vi "SUB_SFCS_SEND_RFPI_IPEI_INFO.vi"(0 "URL":string, 1 "SN":string, 2 "Stage":string, 3 "InfoName":string, 4 "RFID_ID":string="246812345") -> (5 "Pass ?":bool, 6 "All output":string)   [LabVIEW 2011]
uses:
  data/MCSDLL.dll
panel:
  out "OUT1":string
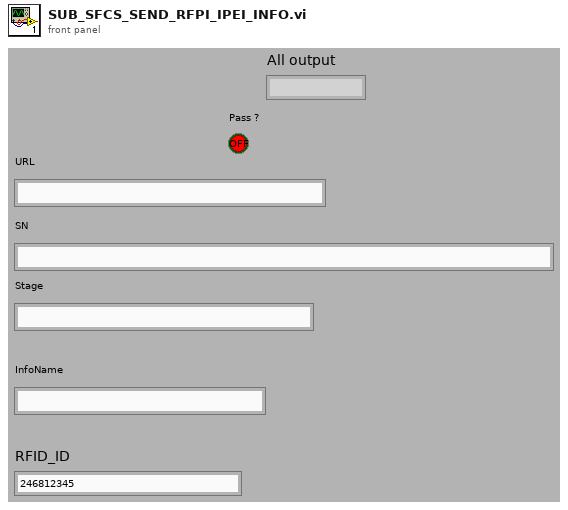
[diagram p1: front panel]
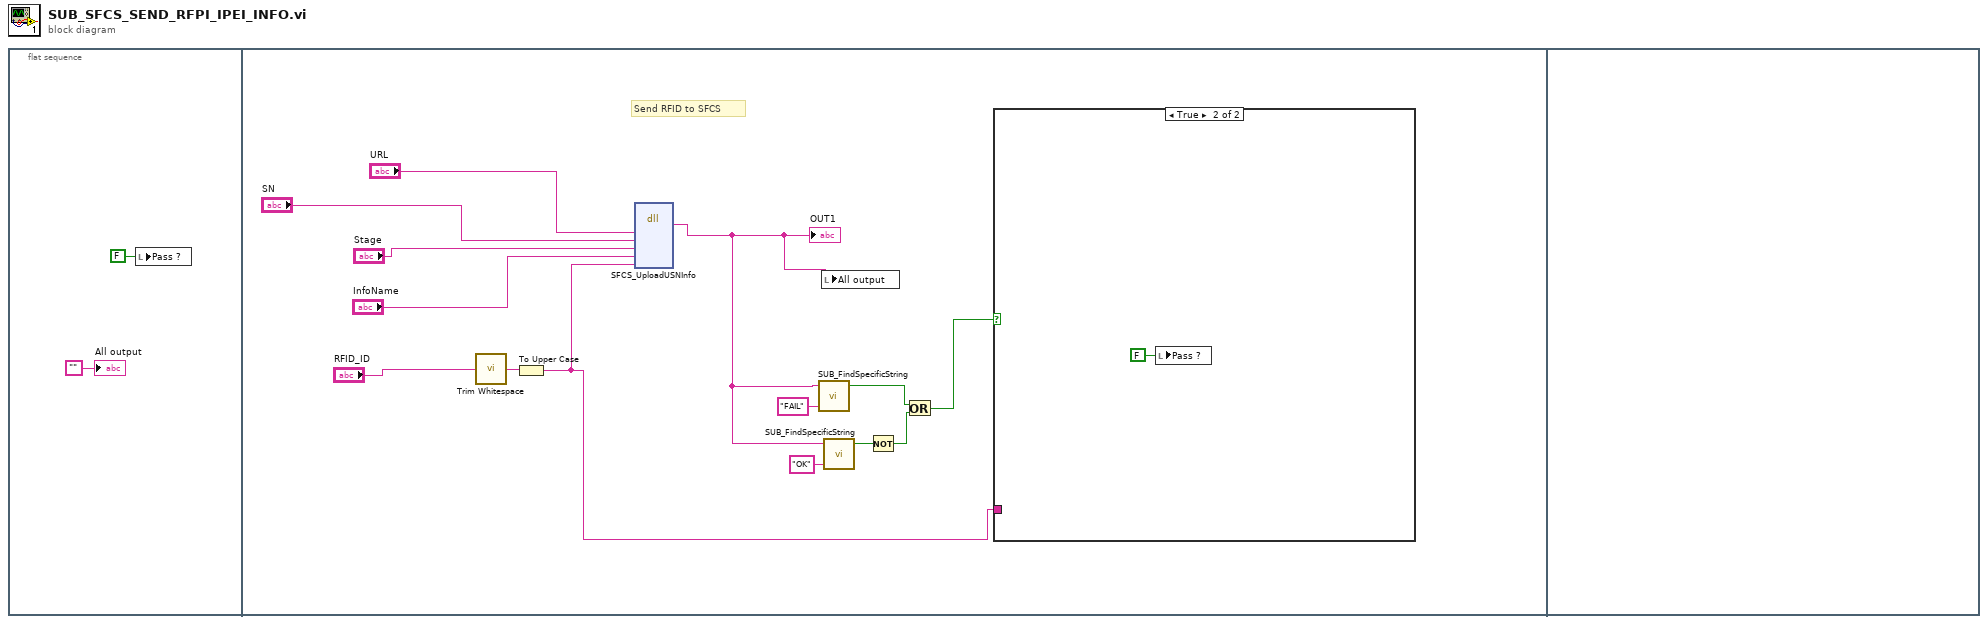
[diagram p0: block diagram]
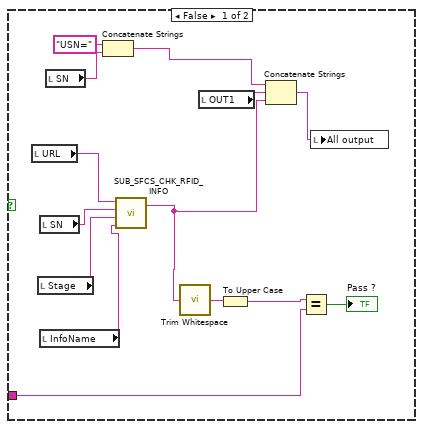
[diagram p2: hidden frame]
diagram:
  n1 = flat-sequence {
    frame #0 {
      n2 = local write "Pass ?"(FALSE ("Pass ?")) -> ()
      "All output" <- ""
    }
    frame #1 {
      # "Send RFID to SFCS"
      n3 = call <vilib>:"Trim Whitespace.vi"("string"="RFID_ID") -> ("trimmed string"=w6:string)  [unwired: 1 in]
      n4 = To Upper Case(1:w6) -> (0:w4:string)
      n5 = dll-call lib="D:/S8300E_Project/data/MCSDLL.dll" fn="SFCS_UploadUSNInfo"("URL"="URL", "SN"="SN", "Stage"="Stage", "InfoName"="InfoName", "RFID_ID"=w4) -> (w3:string)  [unwired: 8 in, 2 out]
      "OUT1" <- w3
      n6 = call "SUB_FindSpecificString.vi"("Find this String"="FAIL", "String data"=w3) -> ("Found"=w10:bool)  [unwired: 2 in, 1 out]
      n7 = local write "All output"(w3) -> ()
      n8 = call "SUB_FindSpecificString.vi"("Find this String"="OK", "String data"=w3) -> ("Found"=w9:bool)  [unwired: 2 in, 1 out]
      n9 = Not(x=w9) -> (.not. x?=w8:bool)
      n10 = Or(x=w10, y=w8) -> (x .or. y?=w7:bool)
      n11 = case shown="True" w7 {
        tunnel: w4 -> [w24 _]
        frame False {
          n12 = local read "URL"() -> (w29:string)
          n13 = local read "Stage"() -> (w27:string)
          n14 = local read "SN"() -> (w28:string)
          n15 = local read "InfoName"() -> (w26:string)
          n16 = local read "SN"() -> (w18:string)
          n17 = Concatenate Strings("USN=" ("string"), w18) -> (w17:string)
          n18 = call "SUB_SFCS_CHK_RFID_INFO.vi"("InfoName"=w26, "Stage"=w27, "SN"=w28, "URL"=w29) -> ("output param"=w21:string)  [unwired: 1 out]
          n19 = call <vilib>:"Trim Whitespace.vi"("string"=w21) -> ("trimmed string"=w25:string)  [unwired: 1 in]
          n20 = local read "OUT1"() -> (w22:string)
          n21 = To Upper Case(1:w25) -> (0:w23:string)
          n22 = Concatenate Strings(w17, w22, w21) -> (w20:string)
          n23 = Equal?(x=w23, y=w24) -> (x = y?=→"Pass ?":bool)
          n24 = local write "All output"(w20) -> ()
        }
        frame True {
          n25 = local write "Pass ?"(FALSE ("Pass ?")) -> ()
        }
      }
    }
    frame #2 {
    }
  }
